vi "Device pattern.vi"(8 "error in (no error)":errorcluster, 10 "Notifiers":T1, 11 "All Message Queue Cluster":T2) -> (0 "error out":errorcluster)   [LabVIEW 2013]
uses:
  Lib QMH/MessageQueues.lvlib
  Device Data.ctl
  Lib QMH/Message Cluster.ctl
  Lib QMH/AllMessageQueue Cluster.ctl
  Lib Notifier/Notifier.ctl
  Lib Notifier/Notifier.lvlib
panel:
  out "Data 1":dbl
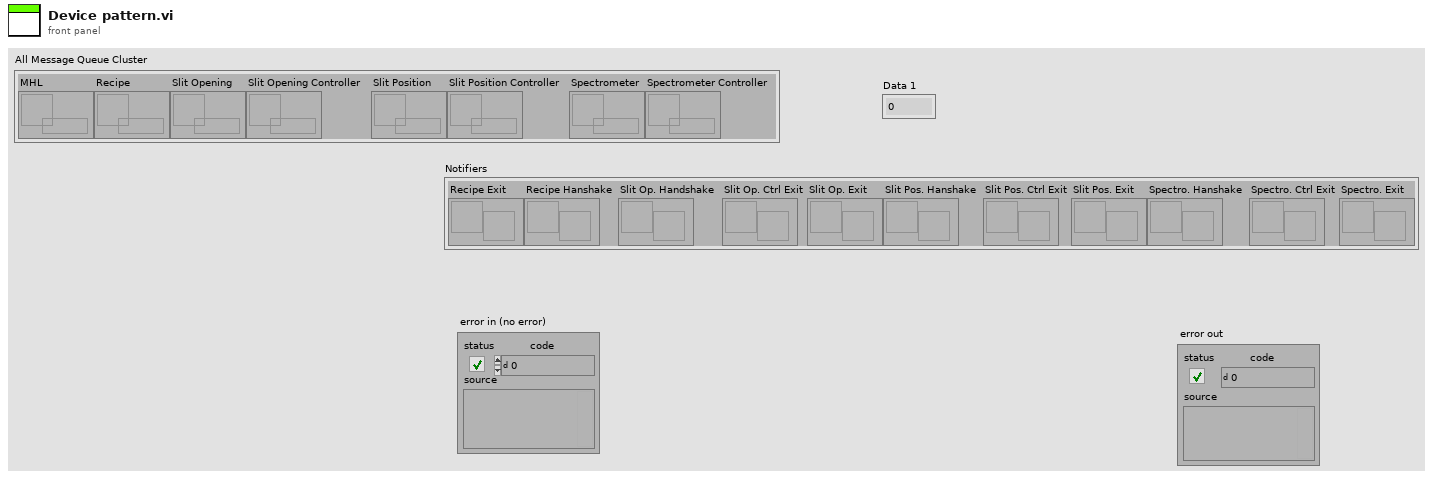
[diagram p1: front panel]
types:
  T1 = typedef "Notifier.lvlib/Notifier.ctl" = cluster{"Recipe Exit":refnum<notifier>, "Recipe Hanshake":refnum<notifier>, "Slit Op. Handshake":refnum<notifier>, "Slit Op. Ctrl Exit":refnum<notifier>, "Slit Op. Exit":refnum<notifier>, "Slit Pos. Hanshake":refnum<notifier>, "Slit Pos. Ctrl Exit":refnum<notifier>, "Slit Pos. Exit":refnum<notifier>, "Spectro. Hanshake":refnum<notifier>, "Spectro. Ctrl Exit":refnum<notifier>, "Spectro. Exit":refnum<notifier>}
  T2 = typedef "MessageQueues.lvlib/AllMessageQueue Cluster.ctl" = cluster{"MHL":refnum<queue>, "Recipe":refnum<queue>, "Slit Opening":refnum<queue>, "Slit Opening Controller":refnum<queue>, "Slit Position":refnum<queue>, "Slit Position Controller":refnum<queue>, "Spectrometer":refnum<queue>, "Spectrometer Controller":refnum<queue>}
  T3 = typedef "Device Data.ctl" = cluster{"Data 1":dbl}
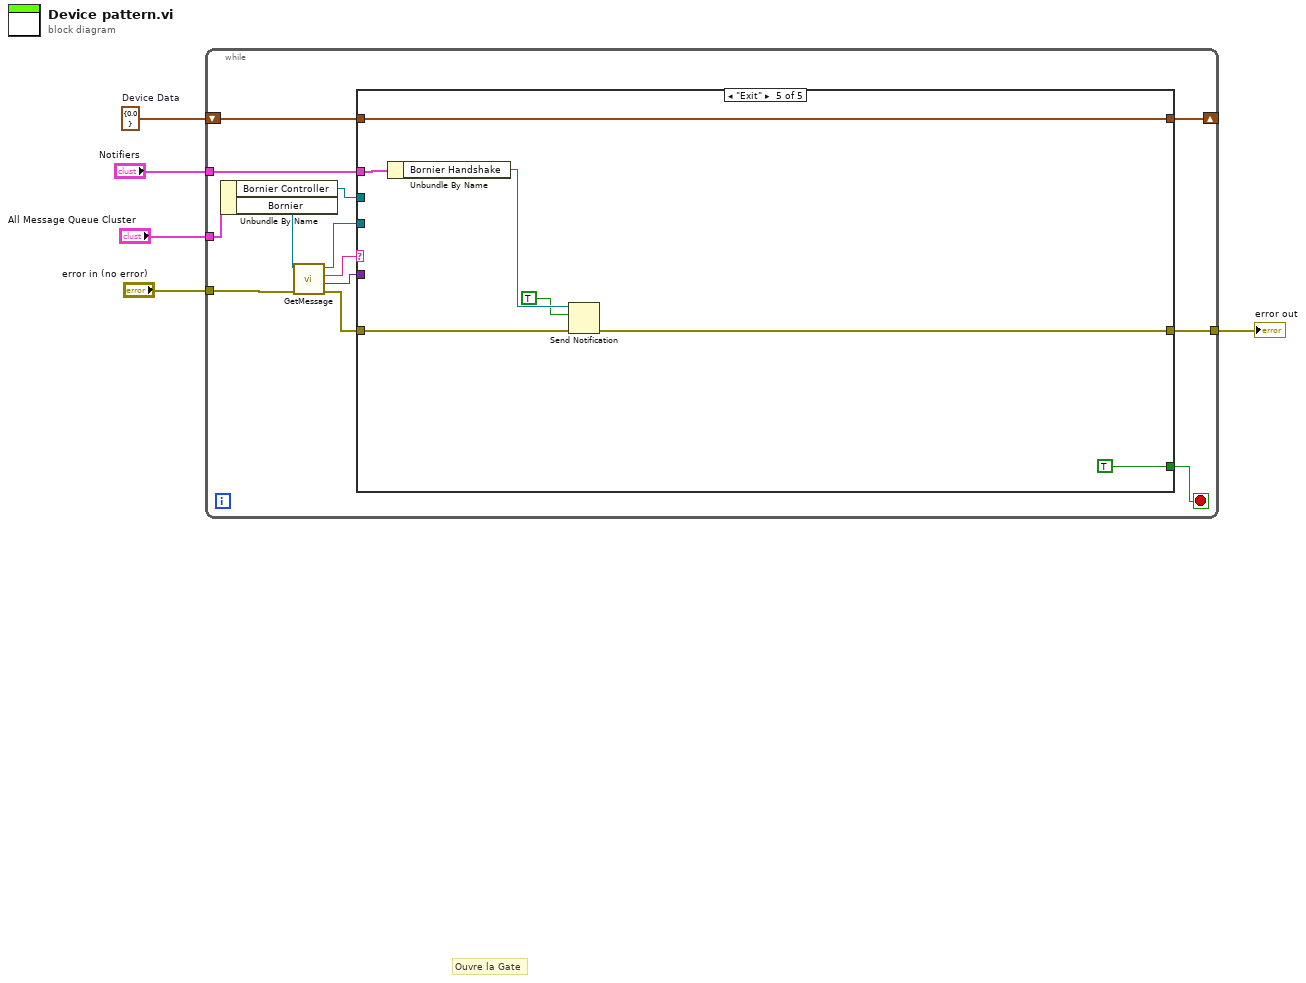
[diagram p0: block diagram]
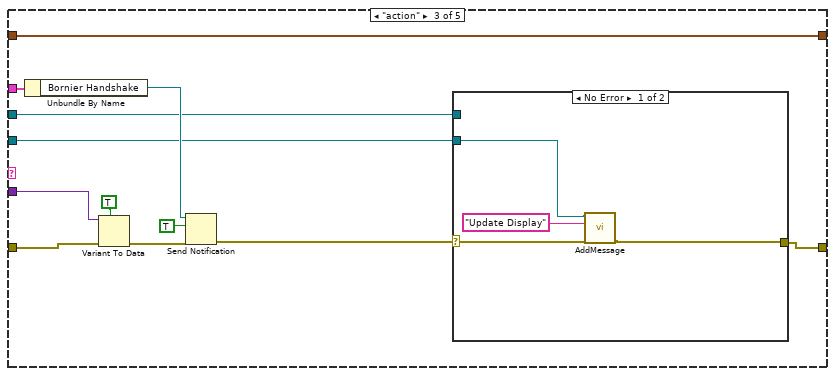
[diagram p4: hidden frame]
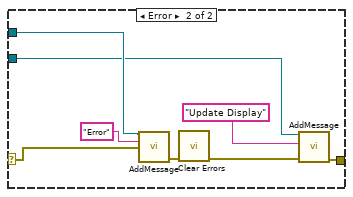
[diagram p5: hidden frame]
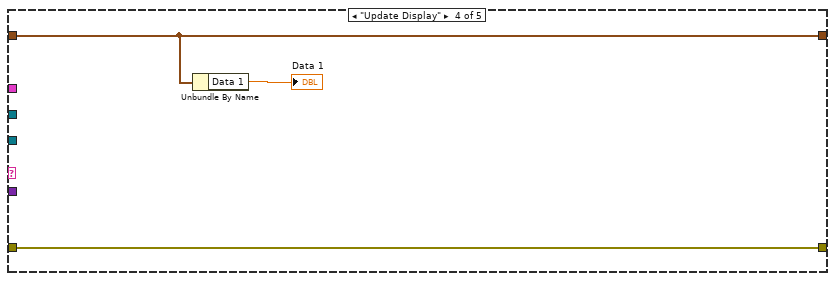
[diagram p6: hidden frame]
diagram:
  w1 = T3 {"Data 1"=0.0}  # Device Data
  # "Ouvre la Gate"
  n1 = while {
    tunnel: "All Message Queue Cluster" -> [w11]
    tunnel: "Notifiers" -> [w18]
    tunnel: "error in (no error)" -> [w12]
    tunnel: [w10] -> w2
    shift-right: [w6] -> _
    shift-left: w1 -> [w7]
    stop <- w8 stop-if-true
    n2 = Unbundle By Name(w11) -> ("Bornier Controller"=w9:refnum<queue>, "Bornier"=w17:refnum<queue>)
    n3 = call "GetMessage.vi"("entrée d'erreur"=w12, "Message queue"=w17) -> ("sortie d'erreur"=w13:errorcluster, "Data"=w14:variant, "Message"=w15:string, "Dup Message Queue"=w16:refnum<queue>)  [unwired: 6 in]
    n4 = case shown="\"Exit\"" w15 {
      tunnel: w18 -> [_ _ w29 _ w55]
      tunnel: w16 -> [_ _ w26 _ _]
      tunnel: w14 -> [_ _ w28 _ _]
      tunnel: w13 -> [w20 w22 w27 w49 w52]
      tunnel: [w20 w22 w25 w49 w51] -> w10
      tunnel: w9 -> [_ _ w24 _ _]
      tunnel: [_ _ _ _ TRUE] -> w8
      tunnel: w7 -> [w19 w21 w23 w47 w50]
      tunnel: [w19 w21 w23 w47 w50] -> w6
      frame Default {
      }
      frame "Initialize" {
      }
      frame "action" {
        n5 = Unbundle By Name(w29) -> ("Bornier Handshake"=w33:refnum<notifier>)
        n6 = Variant To Data(error in=w27, type=TRUE, Variant=w28) -> (error out=w31:errorcluster)  [unwired: 1 out]
        n7 = Send Notification(notification=TRUE, notifier=w33, error in (no error)=w31) -> (error out=w34:errorcluster)  [unwired: 1 out]
        n8 = case shown="No Error" w34 {
          selector: w34 -> [w36 w44]
          tunnel: w26 -> [w38 w42]
          tunnel: [w35 w39] -> w25
          tunnel: w24 -> [_ w46]
          frame No Error {
            n9 = call "AddMessage.vi"("Message queue"=w38, "Message"="Update Display", "entrée d'erreur (pas d'erreur)"=w36) -> ("error out"=w35:errorcluster)  [unwired: 11 in, 1 out]
          }
          frame Error {
            n10 = call "AddMessage.vi"("Message queue"=w46, "Message"="Error", "Data"=w44) -> ("error out"=w43:errorcluster)  [unwired: 11 in, 1 out]
            n11 = call <vilib>:"Clear Errors.vi"("error in (no error)"=w43) -> ("error out"=w40:errorcluster)  [unwired: 6 in]
            n12 = call "AddMessage.vi"("Message queue"=w42, "Message"="Update Display", "entrée d'erreur (pas d'erreur)"=w40) -> ("error out"=w39:errorcluster)  [unwired: 11 in, 1 out]
          }
        }
      }
      frame "Update Display" {
        n13 = Unbundle By Name(w47) -> ("Data 1"=→"Data 1":dbl)
      }
      frame "Exit" {
        n14 = Unbundle By Name(w55) -> ("Bornier Handshake"=w54:refnum<notifier>)
        n15 = Send Notification(notification=TRUE, notifier=w54, error in (no error)=w52) -> (error out=w51:errorcluster)  [unwired: 1 out]
      }
    }
  }
  "error out" <- w2
